vi "Move Focusing Unit.vi"(0 "VISA Resource Name":refnum<visa-resource-name>, 5 "Device Number (1)":i32=1, 7 "Direction (1: Down)":enum16{"Up", "Down"}(ring)=enum."Down", 9 "Step (0.0 um)":dbl format="%.1f", 11 "error in (no error)":errorcluster {"code" format="%.0x"}) -> (4 "VISA Resource Name Out":refnum<visa-resource-name>, 15 "error out":errorcluster {"code" format="%.0x"})   [LabVIEW 2020, in "Olympus IX BX Series.lvlib"]
doc: "Moves the focusing unit."
uses:
  Olympus IX BX Series.lvlib
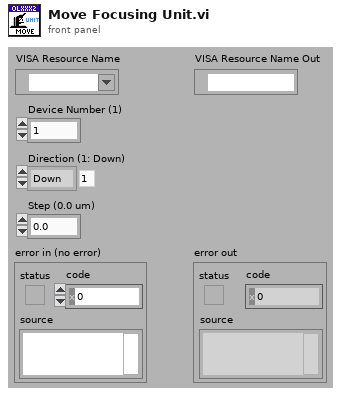
[diagram p1: front panel]
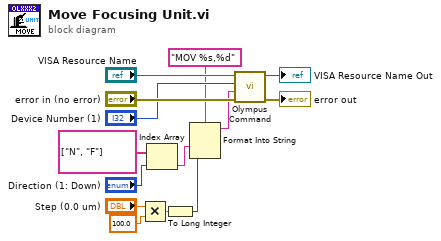
[diagram p0: block diagram]
diagram:
  n1 = Multiply(x="Step (0.0 um)", y=100.0) -> (x*y=w9:dbl)
  n2 = Index Array(array=string[] ["N", "F"], index="Direction (1: Down)") -> (element=w12:string)
  n3 = To Long Integer(number=w9) -> (32bit integer=w8:i32)
  n4 = Format Into String(format string="MOV %s,%d", w12, w8) -> (resulting string=w3:string)  [unwired: 2 in, 1 out]
  n5 = call "Olympus Command.vi"("error in (no error)"="error in (no error)", "Command string"=w3, "Device Number (1)"="Device Number (1)", "VISA Resource Name"="VISA Resource Name") -> ("error out"=→"error out":errorcluster, "VISA Resource Name Out"=→"VISA Resource Name Out":refnum<visa-resource-name>)  [unwired: 5 in, 1 out]
